vi "Read Histogram Measurements.vi"(7 "Analyzer (0: A0)":i32(ring) items=["A0", "A1"], 8 "error in (no error)":errorcluster, 9 "Channel (0: chA)":i32(ring) items=["chA", "chB"], 10 "Measurement (0: Mean)":i32(ring) items=["Mean", "Standard Deviation"], 11 "VISA resource name":refnum<visa-resource-name>) -> (0 "error out":errorcluster, 2 "Histogram Measured Value":dbl, 3 "VISA resource name out":refnum<visa-resource-name>)   [LabVIEW 2014, in "Stanford Research SR1.lvlib"]
doc: "Reads the measurements from the Histogram Digital Generator."
uses:
  Stanford Research SR1.lvlib
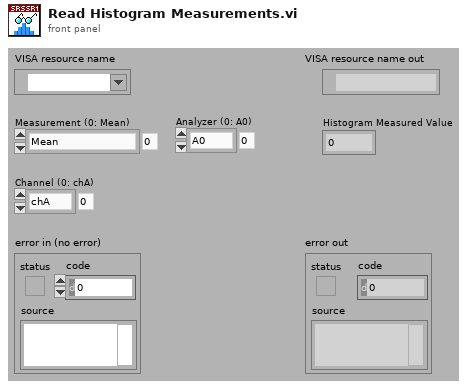
[diagram p1: front panel]
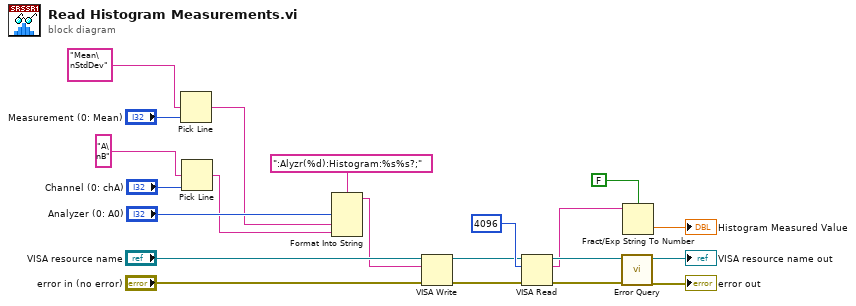
[diagram p0: block diagram]
diagram:
  n1 = Pick Line(multi-line string="Mean\nStdDev", line index="Measurement (0: Mean)") -> (output string=w6:string)  [unwired: 1 in]
  n2 = Pick Line(multi-line string="A\nB", line index="Channel (0: chA)") -> (output string=w5:string)  [unwired: 1 in]
  n3 = Format Into String(format string=":Alyzr(%d):Histogram:%s%s?;", "Analyzer (0: A0)", w6, w5) -> (resulting string=w2:string)  [unwired: 2 in, 1 out]
  n4 = VISA Write(VISA resource name="VISA resource name", write buffer=w2, error in (no error)="error in (no error)") -> (VISA resource name out=w18:refnum<visa-resource-name>, error out=w17:errorcluster)  [unwired: 1 out]
  n5 = VISA Read(VISA resource name=w18, byte count=u32 4096, error in (no error)=w17) -> (VISA resource name out=w16:refnum<visa-resource-name>, read buffer=w4:string, error out=w15:errorcluster)  [unwired: 1 out]
  n6 = call "Error Query.vi"("error in (no error)"=w15, "VISA resource name"=w16) -> ("error out"=→"error out":errorcluster, "VISA resource name out"=→"VISA resource name out":refnum<visa-resource-name>)  [unwired: 6 in, 2 out]
  n7 = Fract/Exp String To Number(use system decimal point (T)=FALSE, string=w4) -> (number=→"Histogram Measured Value":dbl)  [unwired: 2 in, 1 out]
